vi "Python_Interface.vi"() -> (0 "Dission":string)   [LabVIEW 2022 SP3]
panel:
  in  "Light":dbl
  in  "Temperature":dbl
  in  "Water Level":dbl
  in  "pH value":dbl
  in  "Python path":path
  in  "module path":path
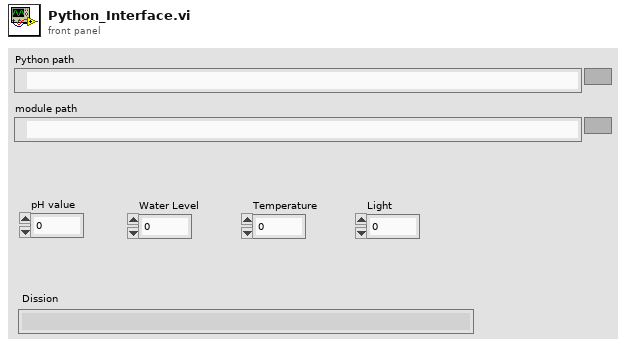
[diagram p1: front panel]
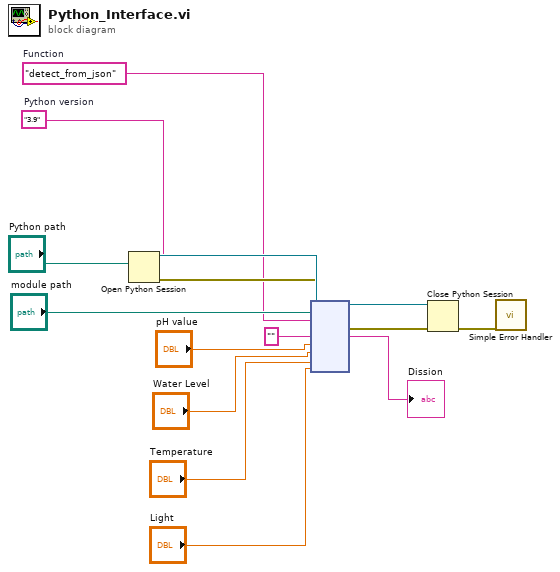
[diagram p0: block diagram]
diagram:
  w5 = "3.9"  # Python version
  w6 = "detect_from_json"  # Function
  n1 = Open Python Session(python version=w5, python path="Python path") -> (session out=w15:refnum<k35>, error out=w10:errorcluster)  [unwired: 1 in]
  n2 = node(w15, "module path", w6, w10, "", "pH value", "Water Level", "Temperature", "Light") -> (w14:refnum<k35>, w13:errorcluster, →"Dission":string)  [unwired: 4 in, 2 out]
  n3 = Close Python Session(session in=w14, error in=w13) -> (11:w11:errorcluster)
  n4 = call <vilib>:"Simple Error Handler.vi"("error in (no error)"=w11) -> ()  [unwired: 4 in, 5 out]
